vi "TwoGenTx_01.vi"() -> ()   [LabVIEW 2021]
uses:
  <vilib>/Analysis/4window.llb/windowTd.ctl
  <vilib>/Analysis/coordinate.llb/Angle Range (Degree).ctl
  <vilib>/Analysis/coordinate.llb/Angle Units.ctl
  <vilib>/Analysis/coordinate.llb/Wrap Angle (scalar).vi
  <vilib>/FPGAPlugInAG/USRP 2945; 2955/niLvFpga_Open_USRP 2945; 2955.vi
  <vilib>/rvi/interface/common/dynamic/niFpgaDynamicAddResources.vi
  <vilib>/FPGAPlugInAG/Dynamic/niLvFpga_Download_Dynamic.vi
  <vilib>/FPGAPlugInAG/Dynamic/niLvFpga_Run_Dynamic.vi
  <vilib>/Utility/error.llb/Error Cluster From Error Code.vi
  <vilib>/rvi/errors/niLvFpgaAdjustHostInterfaceError.vi
  <instrlib>/_niInstr/DSP/v1/FPGA/Public/Sub VIs/Data Conversion/U32 to IQ - 1 spc - S18.1.vi
  <vilib>/measure/maspectr.llb/FFT Spectrum (Mag-Phase) for 1 Chan (CDB).vi
  <vilib>/FPGAPlugInAG/Dynamic/niLvFpga_Close_Dynamic.vi
  <vilib>/rvi/interface/nirviOpenFPGA/nirviOpenFPGA.xnode
  FPGA Bitfiles/usrp2955simpleus_USRP2945;2955_Streaming2955sim_jTXLwECPIws.lvbitx
  <vilib>/rvi/interface/nirviMethod/nirviMethod.xnode
  <vilib>/rvi/interface/nirviReadWriteControl/nirviReadWriteControl.xnode
  <vilib>/rvi/interface/nirviCloseFPGA/nirviCloseFPGA.xnode
  <instrlib>/niUsrpRio/Config/v1/Host/niUsrpRio Config v1 Host.lvlib
  <vilib>/FPGAPlugInAG/Dynamic/niLvFpga_ReadFifo_Dynamic.vi
  <vilib>/rvi/errors/niLvFpgaMergeErrorWithErrorCode.vi
  <instrlib>/_niInstr/DSP/v1/FPGA/niInstr DSP v1 FPGA.lvlib
  <vilib>/Analysis/NI_AALPro.lvlib
  <vilib>/measure/NI_MAPro.lvlib
  <vilib>/Analysis/NI_AAL_Angle.lvlib
  NiFpgaLv.dll
  <vilib>/rvi/interface/Simulation/niFpgaSimulationCallBeginRW.vi
panel:
  in  "cal phase (deg)":dbl[](array[numeric])
  out "phase":dbl[](array[numeric])
  out "scop":dbl[][](graph)
  out "sync error":u32
  out "data sent":u32
  in  "output sample rate":dbl format="%#_6p"
  in  "frequency shift":dbl format="%#_6p"
  out "number of overflows":u64[](array[numeric])
  out "lost sampels":u32
  in  "reset":bool
  out "spectrum":cluster{"f0":dbl, "df":dbl, "magnitude":dbl[]}[](graph)
  in  "WR":bool
  out "error out":errorcluster
  in  "stop":bool
  in  "gain 0":dbl=-20.0 format="%#_6p"
  in  "Tx. frequency 0":dbl=200000000.0 format="%#_6p"
  # "10nSec"
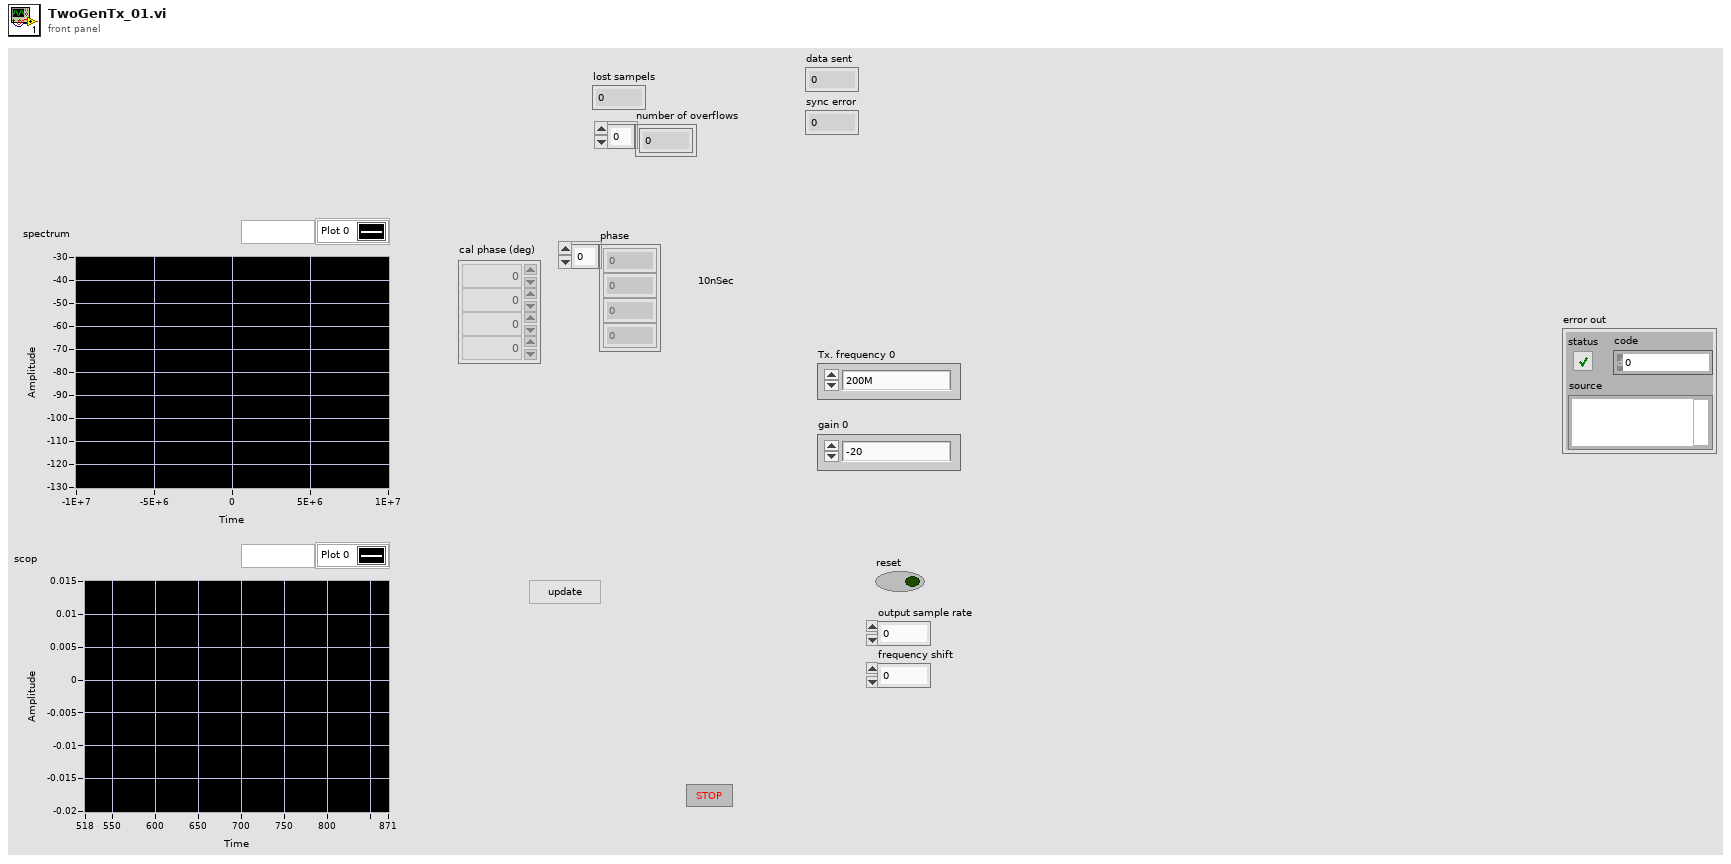
[diagram p1: front panel]
types:
  T1 = cluster{"daughterboard 0 lo configuration":enum16{"Independent", "Import", "Shared and Export", "Reimport", "Shared"}, "daughterboard 1 lo configuration":enum16{"Independent", "Import", "Shared and Export", "Reimport", "Shared"}}
  T2 = typedef "niUsrpRio Config v1 Host.lvlib/niUsrpRio Session.ctl" = cluster{"FPGA Interface":refnum<k20>, "RIO Interface Number":u32, "Data Clock Rate":u32, "FPGA Data Clock Rate":u32, "Global Settings Register Bus":T3, "Radio 0 Settings Register Bus":T3, "Radio 1 Settings Register Bus":T3, "Radio Settings Bus Semaphore":T4, "DB Queues":T5[], "Characterization Data Valid?":bool, "EEPROM Header":T6, "Device Data Header":T7, "EEPROM Characterization Header":T8, "Characterization Data":T9[], "FPGA Current Version":u32, "FPGA Oldest Compatible Version":u32, "Fixed Logic Current Version":u32, "Fixed Logic Oldest Compatible Version":u32, "FPGA Radio Settings Bus Current Version":u32, "FPGA Radio Settings Bus Oldest Compatible Version":u32, "FPGA Board Config Current Version":u32, "FPGA Board Config Oldest Compatible Version":u32, "Daughterboard Clock Rate":u32, "daughterboard configuration session handles":u64[]}
  T3 = typedef "niInstr Register Bus v0 Host.lvlib/Register Bus Session.ctl" = refnum<queue>
  T4 = typedef "Semaphore RefNum" = refnum<k1>
  T5 = typedef "niUsrpRio Config v1 Host.lvlib/DB Queue Reference.ctl" = refnum<queue>
  T6 = typedef "niUsrpRio Config v1 Host.lvlib/EEPROM Header.ctl" = cluster{"Checksum":u32, "Product Code":u16, "Hardware Current Version":u16, "Hardware Oldest Compatible Version":u16, "EEPROM Map Current Version":u16, "EEPROM Map Oldest Compatible Version":u16, "User Password":string, "Pointer to Factory Header":u32, "Pointer to User Header":u32, "Recommended Interval":u16, "Number of Reserved Bytes":i32, "Number of Daughterboards":u8, "Daughterboard IDs":u16[], "Daughterboard Serial Numbers":string[]}
  T7 = typedef "niUsrpRio Config v1 Host.lvlib/EEPROM Device Data Header.ctl" = cluster{"Checksum":u32, "Number of Channels":u8, "Number of Gain Settings":u16[], "Pointer to Characterization Data":u32[], "Number of Reserved Bytes":i32, "Number of Frequencies":u16[]}
  T8 = typedef "niUsrpRio Config v1 Host.lvlib/EEPROM Characterization Header.ctl" = cluster{"Checksum":u32, "Date":timestamp, "Temperature":sgl, "Misc. Info":string, "Pointer to Device Data Header":u32, "Number of Reserved Bytes":i32}
  T9 = typedef "niUsrpRio Config v1 Host.lvlib/Characterization Data.ctl" = cluster{"Gains[dB]":dbl[], "Frequencies [Hz]":dbl[], "IQ Imbalance Table":T10[], "Measured Gains[dB]":dbl[][]}
  T10 = typedef "niUsrpRio Config v1 Host.lvlib/IQ Imbalance.ctl" = cluster{"Gain Imbalance [linear]":dbl, "Phase Imbalance [radians]":dbl, "Offset":cdb}
  T11 = cluster{"output sample rate":fxp<+,48,1>, "delay":fxp<+/-,16,0>, "frequency shift":fxp<+/-,48,0>, "phase":fxp<+/-,21,0>}
  T12 = cluster{"dB On (F)":bool, "unwrap phase (F)":bool, "convert to degree (F)":bool}
  T13 = cluster{"output sample rate":fxp<+,48,1>, "delay":fxp<+/-,16,0>, "frequency shift":fxp<+/-,48,0>, "phase":fxp<+/-,21,0>}[]
  T14 = typedef "NI_AAL_Angle.lvlib/Angle Units.ctl" = i32
  T15 = typedef "NI_AAL_Angle.lvlib/Angle Range (Degree).ctl" = u16
  T16 = typedef "niInstr DSP v1 Shared.lvlib/IQ Data.ctl" = cluster{"I":fxp<+/-,18,1>, "Q":fxp<+/-,18,1>, "overflow":bool}
  T17 = typedef "NI_AALPro.lvlib/windowTd.ctl" = u32
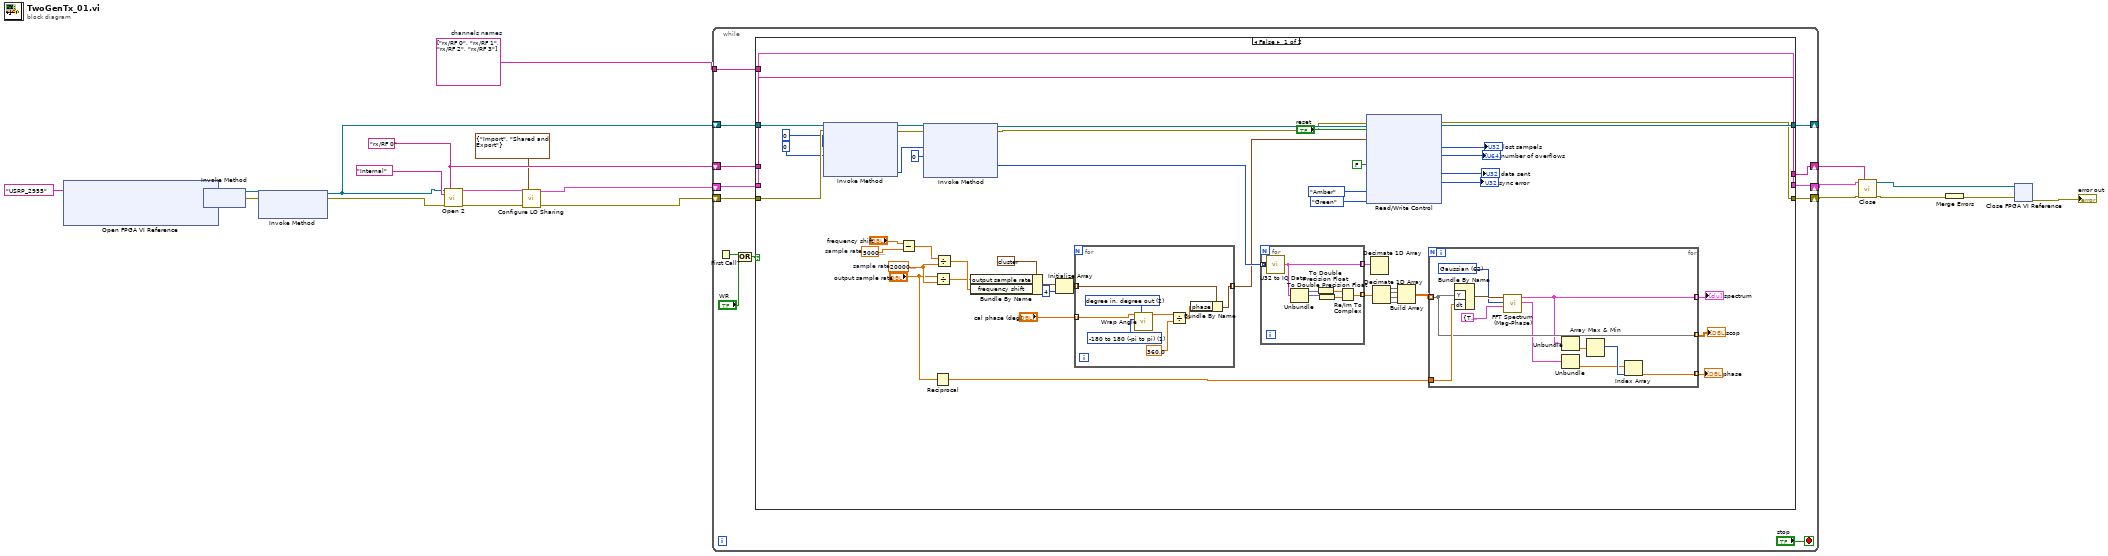
[diagram p0: block diagram]
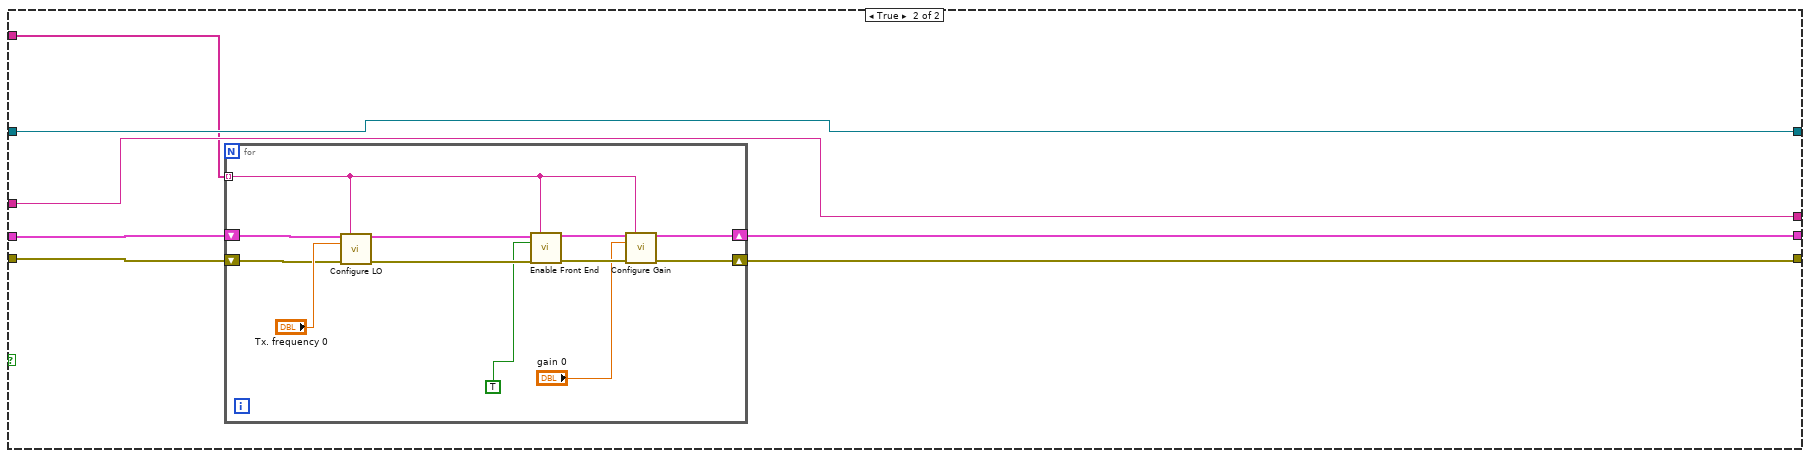
[diagram p2: hidden frame]
diagram:
  w3 = string[] ["rx/RF 0", "rx/RF 1", "rx/RF 2", "rx/RF 3"]  # channels names
  w16 = "rx/RF 0" ("scope")
  n1 = xnode "Open FPGA VI Reference"("resource name"=tag "USRP_2955") -> ("FPGA VI Reference Out"=w19:refnum<k20>, "error out"=w18:errorcluster)  [unwired: 1 in]
  n2 = xnode "Invoke Method"("FPGA VI Reference In"=w19, "error in"=w18) -> ("FPGA VI Reference Out"=w22:refnum<k20>, "error out"=w21:errorcluster)
  n3 = xnode "Invoke Method"("FPGA VI Reference In"=w22, "error in"=w21) -> ("FPGA VI Reference Out"=w14:refnum<k20>, "error out"=w8:errorcluster)  [unwired: 1 in]
  n4 = call <instrlib>:"Open 2.vi"("fpga ref"=w14, "scope"=w16, "Reference Frequency Source"="Internal", "error in"=w8) -> ("niUsrpRio Session (out)"=w7:T2, "error out"=w6:errorcluster)  [unwired: 10 in]
  n5 = call "Configure LO Sharing.vi"("niUsrpRio Session in"=w7, "lo config"=T1 {"daughterboard 0 lo configuration"=enum."Import", "daughterboard 1 lo configuration"=enum."Shared and Export"}, "error in"=w6) -> ("niUsrpRio Session out"=w5:T2, "error out"=w4:errorcluster)  [unwired: 11 in]
  n6 = while {
    shift-right: [w30] -> w12
    shift-left: w4 -> [w34]
    shift-right: [w32] -> w15
    shift-left: w5 -> [w35]
    shift-right: [w31] -> _
    shift-left: w14 -> [w33]
    shift-right: [w27] -> w13
    shift-left: w16 -> [w28]
    tunnel: w3 -> [w23]
    stop <- "stop" stop-if-true
    n7 = First Call?() -> (First Call?: T/F=w25:bool)
    n8 = Or(x=w25, y="WR") -> (x .or. y?=w26:bool)
    n9 = case shown="False" w26 {
      tunnel: w35 -> [w81 w113]
      tunnel: w34 -> [w79 w112]
      tunnel: w33 -> [w80 w111]
      tunnel: [w81 w115] -> w32
      tunnel: [w76 w111] -> w31
      tunnel: [w75 w114] -> w30
      tunnel: w28 -> [w82 w110]
      tunnel: [w82 w110] -> w27
      tunnel: w23 -> [_ w109]
      frame False {
        w41 = 50000000.0  # sample rate
        w60 = 200000000.0  # sample rate
        n10 = xnode "Invoke Method"("FPGA VI Reference In"=w80, "error in"=w79, "Number of Elements"=u32 0, "Timeout (ms)"=0) -> ("FPGA VI Reference Out"=w49:refnum<k20>, "error out"=w50:errorcluster, "Elements Remaining"=w52:u32)  [unwired: 1 out]
        n11 = Subtract(x="frequency shift", y=w41) -> (x-y=w40:dbl)
        n12 = xnode "Invoke Method"("FPGA VI Reference In"=w49, "error in"=w50, "Number of Elements"=w52, "Timeout (ms)"=0) -> ("FPGA VI Reference Out"=w48:refnum<k20>, "error out"=w47:errorcluster, "Data"=w45:u32[])  [unwired: 1 out]
        n13 = Reciprocal(x="output sample rate") -> (1/x=w55:dbl)
        n14 = Divide(x="output sample rate", y=w60) -> (x/y=w59:dbl)
        n15 = Divide(x=w40, y=w60) -> (x/y=w61:dbl)
        n16 = Bundle By Name(cluster=T11 {"output sample rate"=0.0, "delay"=0.0, "frequency shift"=0.0, "phase"=0.0} ("DSP params"), "output sample rate"=w59, "frequency shift"=w61) -> (w62:T11)
        n17 = Initialize Array(w62, 4 ("dimension size")) -> (w38:T13)
        n18 = for {
          tunnel: w38 -> [w90] mode=indexing
          tunnel: [w89] -> w37 mode=indexing
          tunnel: "cal phase (deg)" -> [w85] mode=indexing
          w83 = T14 2 items=["radian in, radian out", "radian in, degree out", "degree in, degree out", "degree in, radian out"] ("angle units")
          w86 = T15 1 items=["none", "-180 to 180 (-pi to pi)", "0 to 360 (0 to 2pi)"] ("angle range")
          n19 = call-poly <vilib>:"Wrap Angle.vi"("angle units"=w83, "angle range"=w86, "angle in"=w85) -> ("angle out"=w84:dbl)  [unwired: 7 in, 1 out]
          n20 = Divide(x=w84, y=360.0) -> (x/y=w88:dbl)
          n21 = Bundle By Name(cluster=w90, "phase"=w88) -> (w89:T11)
        }
        n22 = for {
          tunnel: w45 -> [w108] mode=indexing
          tunnel: [w107] -> w69 mode=indexing
          tunnel: [w106] -> w74 mode=indexing
          n23 = call-poly <instrlib>:"U32 to IQ Data.vi"("U32 data"=w108) -> ("IQ data"=w107:T16)  [unwired: 14 in]
          n24 = Unbundle(w107) -> ("I"=w105:fxp<+/-,18,1>, "Q"=w104:fxp<+/-,18,1>)  [unwired: 1 out]
          n25 = To Double Precision Float(number=w105) -> (double precision float=w103:dbl)
          n26 = To Double Precision Float(number=w104) -> (double precision float=w102:dbl)
          n27 = Re/Im To Complex(1:w102, 2:w103) -> (0:w106:cdb)
        }
        n28 = xnode "Read/Write Control"("FPGA VI Reference In"=w48, "error in"=w47, "reset"="reset", "DSP params"=w37, "reset"=FALSE, "LED/RF /RX1"=enum8{"Off", "Green", "Red", "Amber"}."Amber", "LED/RF /RX2"=enum8{"Off", "Green"}."Green") -> ("FPGA VI Reference Out"=w76:refnum<k20>, "error out"=w75:errorcluster, "lost sampels"=→"lost sampels":u32, "number of overflows"=→"number of overflows":u64[], "data sent"=→"data sent":u32, "sync error"=→"sync error":u32)
        n29 = Decimate 1D Array(w69) -> ()  [unwired: 4 out]
        n30 = Decimate 1D Array(w74) -> (w70:cdb[], w71:cdb[], w72:cdb[], w73:cdb[])
        n31 = Build Array(w70, w71, w72, w73) -> (w58:cdb[][])
        n32 = for {
          tunnel: w58 -> [w98] mode=indexing
          tunnel: [w96] -> w57 mode=indexing
          tunnel: w55 -> [w100]
          tunnel: [w98] -> w46 mode=indexing
          tunnel: [w91] -> w39 mode=indexing
          w99 = T17 62 items=["Rectangle"=0, "Hanning"=1, "Hamming"=2, "Blackman-Harris"=3, "Exact Blackman"=4, "Blackman"=5, "Flat Top"=6, "4 Term B-Harris "=7, "7 Term B-Harris"=8, "Low Sidelobe"=9, "Blackman Nuttall"=11, "Triangle"=30, "Bartlett-Hanning"=31, "Bohman"=32, "Parzen"=33, "Welch"=34, "Kaiser"=60, "Dolph-Chebyshev"=61, "Gaussian"=62] ("window")
          n33 = Bundle By Name("Y"=w98, "dt"=w100) -> (w101:waveform(cdb))  [unwired: 1 in]
          n34 = call-poly <vilib>:"FFT Spectrum (Mag-Phase).vi"("view"=T12 {"dB On (F)"=TRUE, "unwrap phase (F)"=FALSE, "convert to degree (F)"=TRUE}, "window"=w99, "time signal"=w101) -> ("phase"=w93:cluster{"f0":dbl, "df":dbl, "phase":dbl[]}, "magnitude"=w96:cluster{"f0":dbl, "df":dbl, "magnitude":dbl[]})  [unwired: 4 in, 3 out]
          n35 = Unbundle(w96) -> ("magnitude"=w95:dbl[])  [unwired: 2 out]
          n36 = Unbundle(w93) -> ("phase"=w92:dbl[])  [unwired: 2 out]
          n37 = Array Max & Min(array=w95) -> (max index (indices)=w94:i32)  [unwired: 3 out]
          n38 = Index Array(array=w92, index=w94) -> (element=w91:dbl)
        }
        "spectrum" <- w57
        "scop" <- w46
        "phase" <- w39
      }
      frame True {
        n39 = for {
          shift-right: [w121] -> w115
          shift-left: w113 -> [w118]
          shift-right: [w120] -> w114
          shift-left: w112 -> [w117]
          tunnel: w109 -> [w116] mode=indexing
          n40 = call <instrlib>:"Configure LO.vi"("niUsrpRio Session"=w118, "scope"=w116, "frequency"="Tx. frequency 0", "error in"=w117) -> ("niUsrpRio Session (out)"=w127:T2, "error out"=w126:errorcluster)  [unwired: 8 in, 2 out]
          n41 = call <instrlib>:"Enable Front End.vi"("niUsrpRio Session"=w127, "scope"=w116, "enable"=TRUE ("enable 0 2"), "error in"=w126) -> ("niUsrpRio Session (out)"=w125:T2, "error out"=w124:errorcluster)  [unwired: 10 in]
          n42 = call <instrlib>:"Configure Gain.vi"("niUsrpRio Session"=w125, "scope"=w116, "gain"="gain 0", "error in"=w124) -> ("niUsrpRio Session (out)"=w121:T2, "error out"=w120:errorcluster)  [unwired: 9 in, 1 out]
        }
      }
    }
  }
  n43 = call <instrlib>:"Close.vi"("niUsrpRio Session"=w15, "scope"=w13, "error in"=w12) -> ("fpga ref (out)"=w1:refnum<k20>, "error out"=w11:errorcluster)  [unwired: 11 in]
  n44 = Merge Errors(w11) -> (w10:errorcluster)
  n45 = xnode "Close FPGA VI Reference"("FPGA VI Reference In"=w1, "error in"=w10) -> ("error out"=→"error out":errorcluster)
